vi "General_Monitoring_rt.vi"() -> ()   [LabVIEW 2014]
uses:
  <vilib>/Utility/RT CPU Load.ctl
  <vilib>/Platform/TimedLoop/XDataNode/timing_clust.ctl
  <vilib>/Platform/TimedLoop/XDataNode/nitl_modes.ctl
  <vilib>/Platform/TimedLoop/XDataNode/wakeup.ctl
  <vilib>/platform/TimedLoop/XDataNode/XDataNode.xnode
  <vilib>/Platform/TimedLoop/XDataNode/XDNodeRunTimeDep.lvlib
  <vilib>/NI_Real-Time Target Support.lvlib
panel:
  out "Disk Space Used %":dbl
  out "Synced?":bool
  out "Clock_ID":string
  out "AI0":dbl
  out "CPU Load Total":dbl
  out "CPU loads":T1[](array[typedef]) {"ISR (%)" format="%#.2f"; "Idle (%)" format="%#.2f"; "Background (%)" format="%#.2f"; "Normal (%)" format="%#.2f"; "Above Normal (%)" format="%#.2f"; "High (%)" format="%#.2g"; "Timed Structures (%)" format="%#.2g"; "Time Critical (%)" format="%#.2g"; "Total (%)" format="%#.2g"}
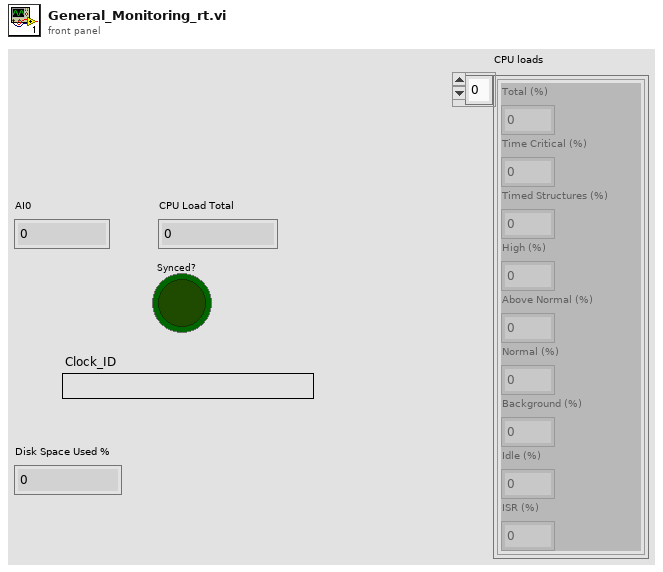
[diagram p1: front panel]
types:
  T1 = typedef "NI_Real-Time Target Support.lvlib/RT CPU Load.ctl" = cluster{"Total (%)":dbl, "Time Critical (%)":dbl, "Timed Structures (%)":dbl, "High (%)":dbl, "Above Normal (%)":dbl, "Normal (%)":dbl, "Background (%)":dbl, "Idle (%)":dbl, "ISR (%)":dbl}
  T2 = typedef "XDNodeRunTimeDep.lvlib/timing_clust.ctl" = cluster{"Expected End [f-1]":u64, "Actual End [f-1]":u64, "Finished Late? [f-1]":bool, "Expected End [i-1]":u64, "Actual End [i-1]":u64, "Finished Late? [i-1]":bool, "Expected Start [i]":u64, "Actual Start [i]":u64, "Expected Start [f]":u64, "Actual Start [f]":u64, "Source Name":string, "Structure Name":string, "Period":i64, "Deadline":i64, "Offset":i64, "Start":i64, "Priority":i32, "Timeout":i32, "Mode":T3, "Wakeup Reason":T4, "Error":errorcluster, "Source Type":string, "Secondary Source Type":string, "Global End Time":u64, "Global Start Time":u64, "Frame Duration":u64, "Iteration Duration":u64, "Assigned CPU":i32, "I/O Scan Engine Mode":u32}
  T3 = typedef "XDNodeRunTimeDep.lvlib/nitl_modes.ctl" = enum32{"No Change", "Process missed periods, maintain original phase", "Discard missed periods, maintain original phase", "Process missed periods, ignore original phase", "Discard missed periods, ignore original phase"}
  T4 = typedef "XDNodeRunTimeDep.lvlib/wakeup.ctl" = enum32{"Normal", "Aborted", "Asynchronous wakeup", "Timing source error", "Timed loop error", "Timeout"}
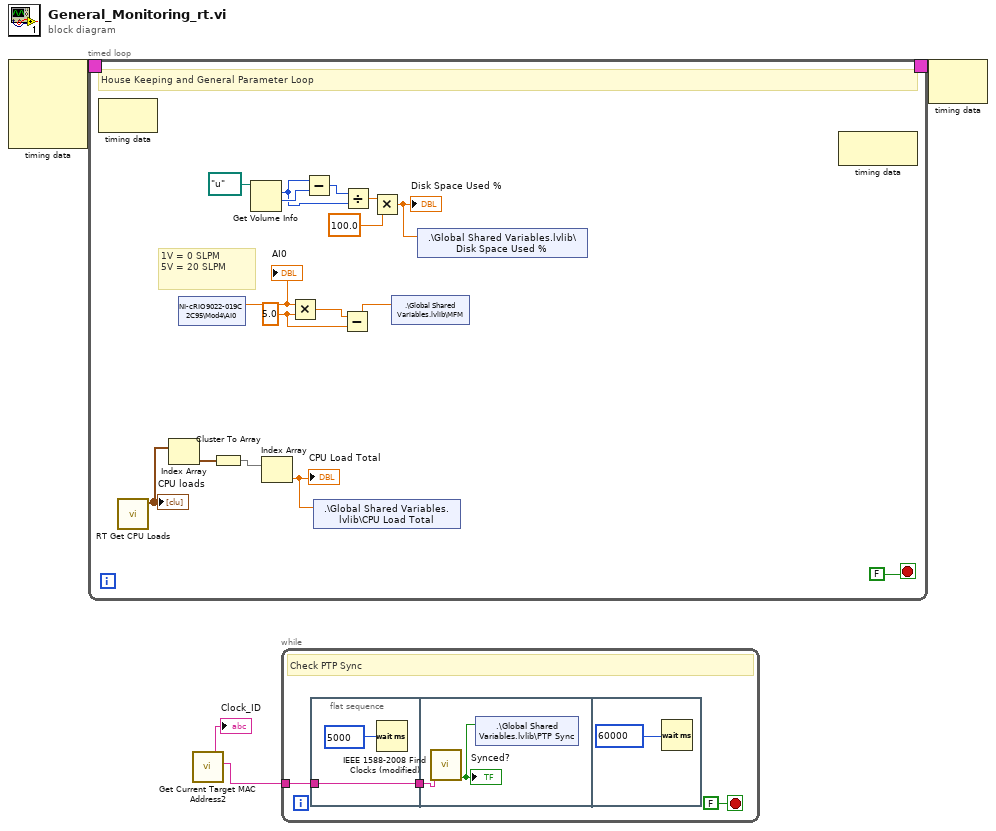
[diagram p0: block diagram]
diagram:
  n1 = node-c288() -> (w3:T2)  [unwired: 4 in]
  n2 = timed-loop {
    timing: w3 -> [_]
    timing-out: [_] -> w2
    stop <- FALSE stop-if-true
    w11 = 5.0 ("y")
    # "1V = 0 SLPM\n5V = 20 SLPM"
    # "House Keeping and General Parameter Loop"
    n3 = node-c288() -> ()  [unwired: 1 in, 1 out]
    n4 = call <vilib>:"RT Get CPU Loads.vi"() -> ("CPU loads"=w19:T1[])  [unwired: 10 in, 1 out]
    "CPU loads" <- w19
    n5 = Index Array(array=w19) -> (element=w18:T1)  [unwired: 1 in]
    n6 = shared-variable "NI-cRIO9022-019C2C95\\Mod4\\AI0"() -> (w14:dbl)  [unwired: 1 in, 1 out]
    "AI0" <- w14
    n7 = Cluster To Array(cluster=w18) -> (array=w16:dbl[])
    n8 = Get Volume Info(11:path "u:/" ("path")) -> (1:w9:i64, 2:w7:i64)  [unwired: 1 in, 4 out]
    n9 = Index Array(array=w16) -> (element=w15:dbl)  [unwired: 1 in]
    "CPU Load Total" <- w15
    n10 = Multiply(x=w14, y=w11) -> (x*y=w12:dbl)
    n11 = Subtract(x=w7, y=w9) -> (x-y=w8:i64)
    n12 = shared-variable ".\\Global Shared Variables.lvlib\\CPU Load Total"(w15) -> ()  [unwired: 1 in, 1 out]
    n13 = Subtract(x=w12, y=w11) -> (x-y=w13:dbl)
    n14 = Divide(x=w8, y=w7) -> (x/y=w6:dbl)
    n15 = Multiply(x=w6, y=100.0) -> (x*y=w4:dbl)
    "Disk Space Used %" <- w4
    n16 = shared-variable ".\\Global Shared Variables.lvlib\\MFM"(w13) -> ()  [unwired: 1 in, 1 out]
    n17 = shared-variable ".\\Global Shared Variables.lvlib\\Disk Space Used %"(w4) -> ()  [unwired: 1 in, 1 out]
    n18 = node-c288() -> ()  [unwired: 1 in, 1 out]
  }
  n19 = call "Get Current Target MAC Address2.vi"() -> ("Clock_ID"=w1:string)  [unwired: 9 in, 2 out]
  "Clock_ID" <- w1
  n20 = while {
    tunnel: w1 -> [w24]
    stop <- FALSE stop-if-true
    # "Check PTP Sync"
    n21 = flat-sequence {
      tunnel: w24 -> [w26]
      tunnel: [w26] -> w23
      tunnel: w23 -> [w28]
      frame #0 {
        n22 = Wait (ms)(milliseconds to wait=u32 5000) -> ()  [unwired: 1 out]
      }
      frame #1 {
        n23 = call "IEEE 1588-2008 Find Clocks (modified).vi"("Clock Id to Verify"=w28) -> ("Synced?"=w27:bool)  [unwired: 10 in]
        "Synced?" <- w27
        n24 = shared-variable ".\\Global Shared Variables.lvlib\\PTP Sync"(w27) -> ()  [unwired: 1 in, 1 out]
      }
      frame #2 {
        n25 = Wait (ms)(milliseconds to wait=u32 60000) -> ()  [unwired: 1 out]
      }
    }
  }
  n26 = node-c288(w2) -> ()  [unwired: 1 out]
